vi "myRIO_BRig_RT_dataCurrent_TpB.vi"() -> (2 "output_TpB":i32)   [LabVIEW 2014]
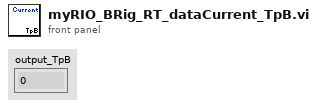
[diagram p1: front panel]
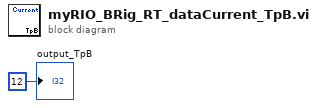
[diagram p0: block diagram]
diagram:
  "output_TpB" <- 12 ("output_iBlock")
